vi "MU Get PRES_POS.vi"(8 "error in (no error)":errorcluster, 11 "handle":u64) -> (0 "error out (no error)":errorcluster, 2 "value":u64, 3 "function return":u32)   [LabVIEW 2017, in "MU_3SL_interface.lvlib"]
uses:
  MU_3SL_interface.lvlib
  lib/MU_3SL_interface.dll
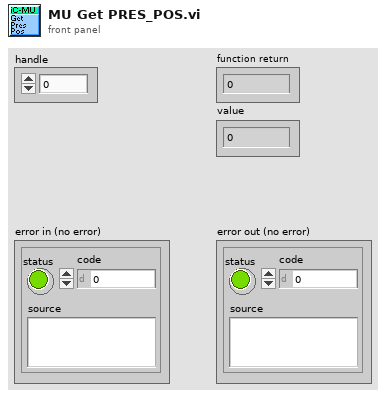
[diagram p1: front panel]
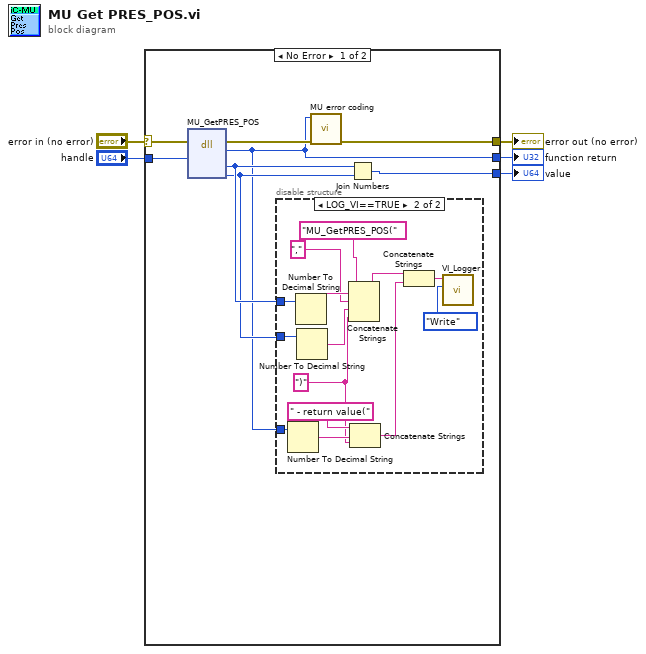
[diagram p0: block diagram]
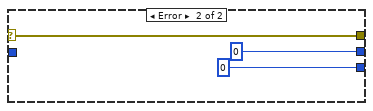
[diagram p3: hidden frame]
diagram:
  n1 = case shown="No Error" "error in (no error)" {
    selector: "error in (no error)" -> [w10 w30]
    tunnel: [w6 u32 0] -> w5
    tunnel: "handle" -> [w13 _]
    tunnel: [w11 w30] -> w3
    tunnel: [w9 u64 0] -> w1
    frame No Error {
      n2 = dll-call lib="C:/Users/bes/AppData/Roaming/work/mu_9so/icsubmodules/soft_mu_3sl_master/lv_interface/lib/MU_3SL_interface**.*" fn="MU_GetPRES_POS"(error in=w10, "handle"=w13) -> (error out=w12:errorcluster, "return type"=w6:u32, "valueHigh"=w8:u32, "valueLow"=w7:u32)  [unwired: 5 in, 1 out]
      n3 = disable-structure shown="LOG_VI==TRUE" {
        disable-tunnel: w6 -> [_ w25]
        disable-tunnel: w8 -> [_ w20]
        disable-tunnel: w7 -> [_ w17]
        frame condition #0 {
        }
        frame condition #1 (active) {
          w14 = ")" ("string")
          n4 = Number To Decimal String(number=w25) -> (decimal integer string=w24:string)  [unwired: 1 in]
          n5 = Number To Decimal String(number=w20) -> (decimal integer string=w19:string)  [unwired: 1 in]
          n6 = Number To Decimal String(number=w17) -> (decimal integer string=w16:string)  [unwired: 1 in]
          n7 = Concatenate Strings("MU_GetPRES_POS(" ("Info in"), w19, "," ("string"), w16, w14) -> (w23:string)
          n8 = Concatenate Strings(" - return value(" ("string"), w24, w14) -> (w22:string)
          n9 = Concatenate Strings(w23, w22) -> (w21:string)
          n10 = call "VI_Logger.vi"("Action (Read)"=enum16{"Write", "Read"}."Write", "Info in"=w21) -> ()  [unwired: 8 in, 2 out]
        }
      }
      n11 = call "MU error coding.vi"("error in (no error)"=w12, "function return in"=w6) -> ("error out"=w11:errorcluster)  [unwired: 9 in]
      n12 = Join Numbers(hi=w8, lo=w7) -> ((hi.lo)=w9:u64)
    }
    frame Error {
    }
  }
  "function return" <- w5
  "error out (no error)" <- w3
  "value" <- w1
